vi "3D Arrow Pad.vi"() -> ()   [LabVIEW 2009]
panel:
  in  "Up":bool
  in  "Left":bool
  in  "Right":bool
  in  "Down":bool
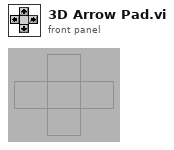
[diagram p1: front panel]
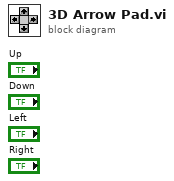
[diagram p0: block diagram]
diagram:
